vi "Create Test GUID.vi"(4 "length":i32) -> (1 "random data":string)   [LabVIEW 2011, in "VITesterUtilities.lvlib"]
doc: "Outputs a <B>random data</B> string of the specified <B>length</B>."
uses:
  Libraries/VITesterUtilities.lvlib
panel:
  # "Copyright © 2006 James Kring, Inc. All rights reserved.\n\nThis library is provided \"AS IS\" , WITHOUT WARRANTIES OR \nCONDITIONS OF ANY KIND, either express or implied.\n\nJames Kring, Inc. -- http://www.jameskring.com"
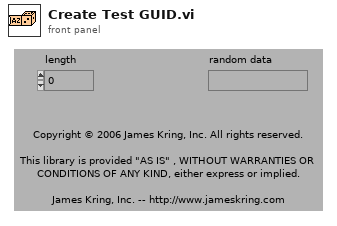
[diagram p1: front panel]
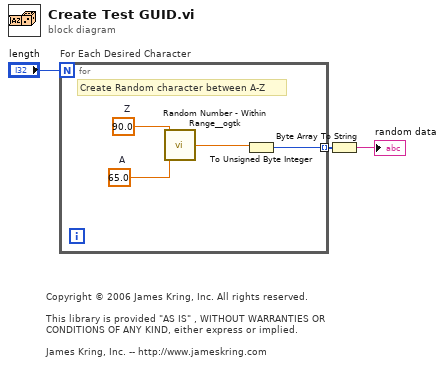
[diagram p0: block diagram]
diagram:
  # "Copyright © 2006 James Kring, Inc. All rights reserved.\n\nThis library is provided \"AS IS\" , WITHOUT WARRANTIES OR \nCONDITIONS OF ANY KIND, either express or implied.\n\nJames Kring, Inc. -- http://www.jameskring.com"
  n1 = for "For Each Desired Character" {
    N: "length" -> [_]
    tunnel: [w7] -> w2 mode=indexing
    w6 = 90.0  # Z
    w5 = 65.0  # A
    # "Create Random character between A-Z"
    n2 = call <userlib>:"Random Number - Within Range__ogtk.vi"("High (1.00)"=w6, "Low (0.00)"=w5) -> ("Random #"=w4:dbl)  [unwired: 3 in]
    n3 = To Unsigned Byte Integer(number=w4) -> (unsigned 8bit integer=w7:u8)
  }
  n4 = Byte Array To String(unsigned byte array=w2) -> (string=→"random data":string)
